vi "Get Tuner Gain.vi"(8 "error in (no error)":errorcluster, 11 "RTL-SDR in":refnum<class "RTL-SDR.lvclass">) -> (0 "error out":errorcluster, 2 "Gain (dB)":dbl, 3 "RTL-SDR out":refnum<class "RTL-SDR.lvclass">)   [LabVIEW 2015, in "RTL-SDR.lvclass"]
uses:
  RTL-SDR.lvclass
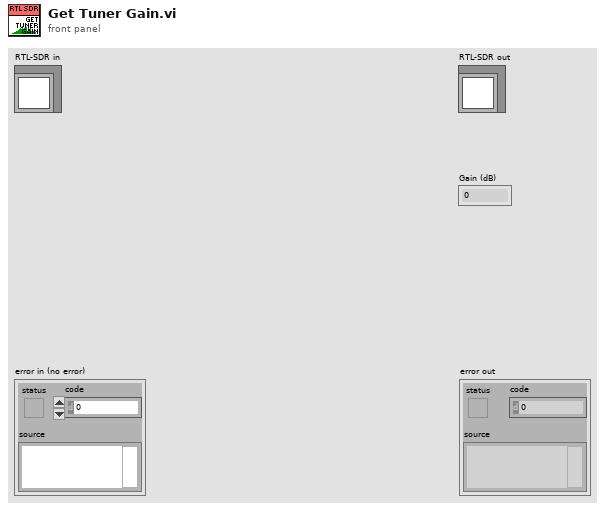
[diagram p1: front panel]
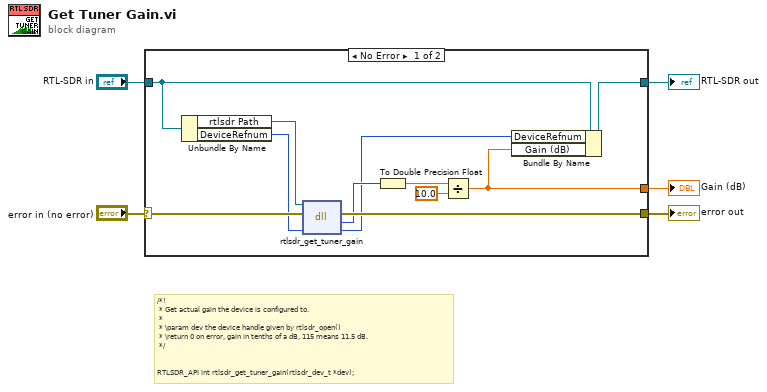
[diagram p0: block diagram]
diagram:
  # "/*!\n * Get actual gain the device is configured to.\n *\n * \\param dev the device handle given by rtlsdr_open()\n * \\return 0 on error, gain in tenths of a dB, 115 means 11.5 dB.\n */\n\n\nRTLSDR_API int rtlsdr_get_tuner_gain(rtlsdr_dev_t *dev);"
  n1 = case shown="No Error" "error in (no error)" {
    selector: "error in (no error)" -> [w16 w18]
    tunnel: [w15 w18] -> w4
    tunnel: [w8 w17] -> w2
    tunnel: "RTL-SDR in" -> [w11 w17]
    tunnel: [w6 _] -> w1
    frame No Error {
      n2 = Unbundle By Name(w11) -> ("rtlsdr Path"=w10:path, "DeviceRefnum"=w9:u64)
      n3 = dll-call lib="C:/Users/Ivan/Desktop/D-23-09-24 (RTL-SDR)/Project (Pelleng-SDR)/RTL-SDR Class/dll/rtlsdr.*" fn="rtlsdr_get_tuner_gain"(path in=w10, error in=w16, "DeviceRefnum"=w9) -> (error out=w15:errorcluster, "Gain"=w12:i32, "DeviceRefnum"=w7:u64)  [unwired: 1 in, 1 out]
      n4 = To Double Precision Float(number=w12) -> (double precision float=w13:dbl)
      n5 = Divide(x=w13, y=10.0) -> (x/y=w6:dbl)
      n6 = Bundle By Name(cluster=w11, "DeviceRefnum"=w7, "Gain (dB)"=w6) -> (w8:refnum<class "RTL-SDR.lvclass">)
    }
    frame Error {
    }
  }
  "error out" <- w4
  "RTL-SDR out" <- w2
  "Gain (dB)" <- w1
